vi "GetValueStringFromColor.vi"(10 "Value Width":enum16{"4-bit", "8-bit"}(ring), 11 "Color":u32(colorbox)) -> (3 "Value String":string)   [LabVIEW 2025, in "ArduinoSerialBling.lvlib"]
uses:
  ArduinoSerialBling.lvlib
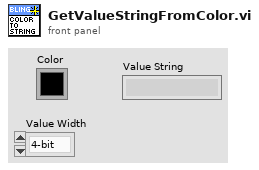
[diagram p1: front panel]
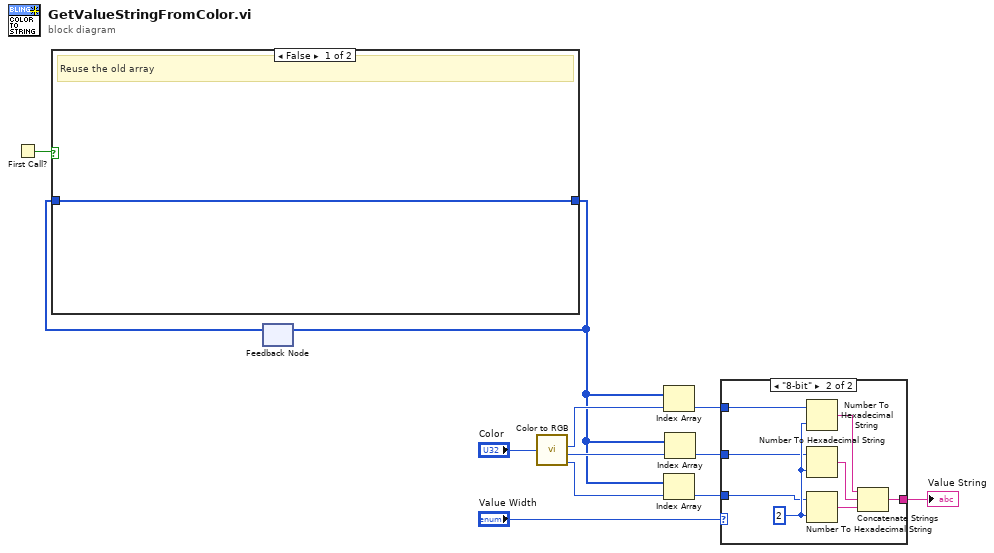
[diagram p0: block diagram]
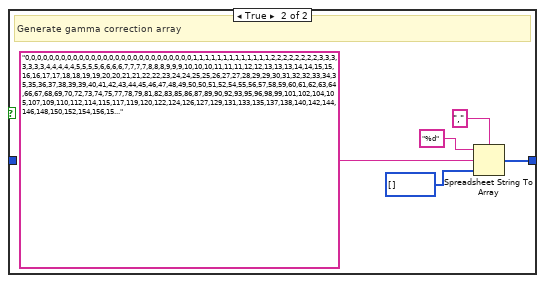
[diagram p2: hidden frame]
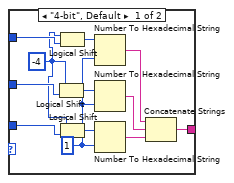
[diagram p3: hidden frame]
diagram:
  n1 = First Call?() -> (First Call?: T/F=w1:bool)
  n2 = feedback #1() -> (w2:u8[])  [unwired: 1 in]
  n3 = case shown="False" w1 {
    tunnel: [w13 w15] -> w3
    tunnel: w2 -> [w13 _]
    frame False {
      # "Reuse the old array"
    }
    frame True {
      # "Generate gamma correction array"
      n4 = Spreadsheet String To Array(delimiter (Tab)=",", format string="%d", spreadsheet string="0,0,0,0,0,0,0,0,0,0,0,0,0,0,0,0,0,0,0,0,0,0,0,0,0,0,0,0,1,1,1,1,1,1,1,1,1,1,1,1,1,2,2,2,2,2,2,2,2,3,3,3,3,3,3,3,4,4,4,4,4,5,5,5,5,6,6,6,6,7,7,7,7,8,8,8,9,9,9,10,10,10,11,11,11,12,12,13,13,13,14,14,15,15,16,16,17,17,18,18,19,19,20,20,21,21,22,22,23,24,24,25,25,26,27,27,28,29,29,30,31,32,32,33,34,35,35,36,37,38,39,39,40,41,42,43,44,45,46,47,48,49,50,50,51,52,54,55,56,57,58,59,60,61,62,63,64,66,67,68,69,70,72,73,74,75,77,78,79,81,82,83,85,86,87,89,90,92,93,95,96,98,99,101,102,104,105,107,109,110,112,114,115,117,119,120,122,124,126,127,129,131,133,135,137,138,140,142,144,146,148,150,152,154,156,158,160,162,164,167,169,171,173,175,177,180,182,184,186,189,191,193,196,198,200,203,205,208,210,213,215,218,220,223,225,228,231,233,236,239,241,244,247,249,252,255", array type (2D Dbl)=u8[] []) -> (array=w15:u8[])
    }
  }
  n5 = feedback-in #1(w3) -> ()
  n6 = call <vilib>:"Color to RGB.vi"("Color"="Color") -> ("R"=w9:u8, "G"=w8:u8, "B"=w7:u8)  [unwired: 1 out]
  n7 = Index Array(array=w3, index=w9) -> (element=w4:u8)
  n8 = Index Array(array=w3, index=w7) -> (element=w6:u8)
  n9 = Index Array(array=w3, index=w8) -> (element=w5:u8)
  n10 = case shown="\"8-bit\"" "Value Width" {
    tunnel: w4 -> [w25 w37]
    tunnel: w5 -> [w20 w36]
    tunnel: w6 -> [w21 w35]
    tunnel: [w26 w31] -> w12
    frame "4-bit", Default {
      w19 = -4
      w30 = i16 1 ("width (-)")
      n11 = Logical Shift(y=w19, x=w20) -> (x << y=w23:u8)
      n12 = Logical Shift(y=w19, x=w25) -> (x << y=w24:u8)
      n13 = Logical Shift(y=w19, x=w21) -> (x << y=w22:u8)
      n14 = Number To Hexadecimal String(1:w30, 2:w24) -> (0:w29:string)
      n15 = Number To Hexadecimal String(1:w30, 2:w23) -> (0:w28:string)
      n16 = Number To Hexadecimal String(1:w30, 2:w22) -> (0:w27:string)
      n17 = Concatenate Strings(w29, w28, w27) -> (w26:string)
    }
    frame "8-bit" {
      w38 = i16 2 ("width (-)")
      n18 = Number To Hexadecimal String(1:w38, 2:w37) -> (0:w34:string)
      n19 = Number To Hexadecimal String(1:w38, 2:w36) -> (0:w33:string)
      n20 = Number To Hexadecimal String(1:w38, 2:w35) -> (0:w32:string)
      n21 = Concatenate Strings(w34, w33, w32) -> (w31:string)
    }
  }
  "Value String" <- w12
